vi "sc5511a_reg_write.vi"(0 "deviceHandle":u32 format="%.0x", 2 "Register":T1(ring), 3 "Data In U64":u64 format="%.0x", 5 "error in":errorcluster) -> (14 "deviceHandle":u32 format="%.0x", 19 "error out":errorcluster)   [LabVIEW 2010]
uses:
  sc5511a_rs232.dll
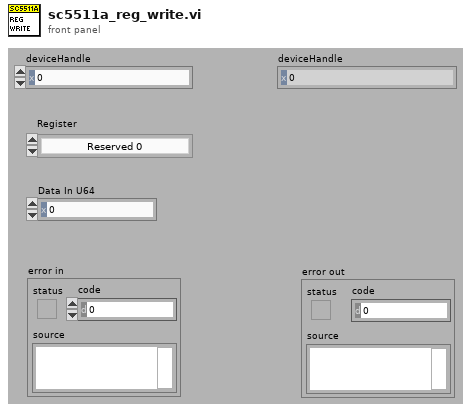
[diagram p1: front panel]
types:
  T1 = enum16{"Reserved 0", "Init", "System Active", "SynthMode", "RF Mode", "List Mode Config", "List Start Freq", "List Stop Freq", "List Step Freq", "List Dwell Time", "List Run Cycles", "Reserved1", "List Buffer Size", "List Buffer Write", "List Buffer to Mem Transfer", "Soft Trigger", "RF Frequency", "RF Level", "RF Enable", "Reserved2", "Auto Level Disable", "ALC Mode", "RF1 Standby", "Reference Setting", "Reference Dac", "ALC Dac", "Reserved3", "Store Default State", "Reserved4", "Reserved5", "RF2 Standby", "RF2 Frequency"}
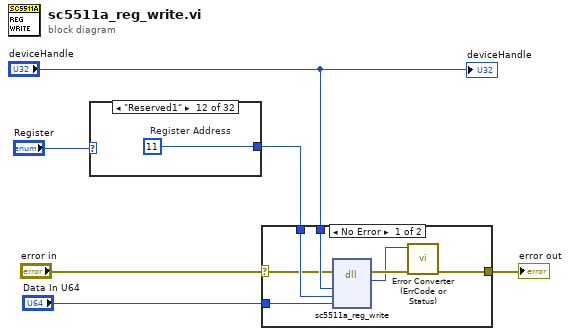
[diagram p0: block diagram]
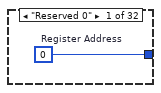
[diagram p2: hidden frame]
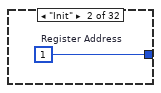
[diagram p3: hidden frame]
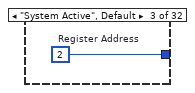
[diagram p4: hidden frame]
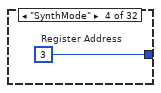
[diagram p5: hidden frame]
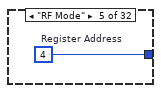
[diagram p6: hidden frame]
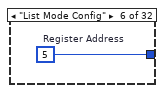
[diagram p7: hidden frame]
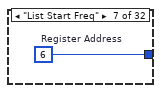
[diagram p8: hidden frame]
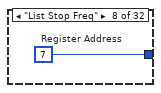
[diagram p9: hidden frame]
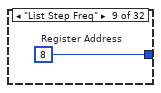
[diagram p10: hidden frame]
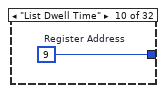
[diagram p11: hidden frame]
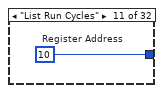
[diagram p12: hidden frame]
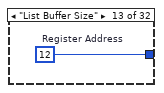
[diagram p13: hidden frame]
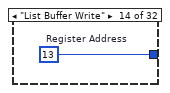
[diagram p14: hidden frame]
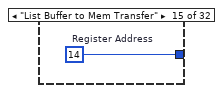
[diagram p15: hidden frame]
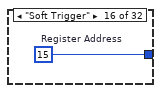
[diagram p16: hidden frame]
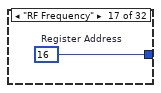
[diagram p17: hidden frame]
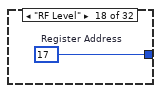
[diagram p18: hidden frame]
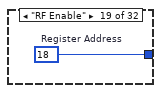
[diagram p19: hidden frame]
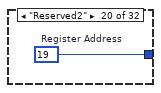
[diagram p20: hidden frame]
diagram:
  n1 = case shown="\"Reserved1\"" "Register" {
    tunnel: [w7 w8 w9 w10 w11 w12 w13 w14 w15 w16 w17 w18 w19 w20 w21 w22 w23 w24 w25 w26 w27 w28 w29 w30 w31 w32 w33 w34 w35 w36 w37 w38] -> w2
    frame "Reserved 0" {
      w7 = u8 0  # Register Address
    }
    frame "Init" {
      w8 = u8 1  # Register Address
    }
    frame "System Active", Default {
      w9 = u8 2  # Register Address
    }
    frame "SynthMode" {
      w10 = u8 3  # Register Address
    }
    frame "RF Mode" {
      w11 = u8 4  # Register Address
    }
    frame "List Mode Config" {
      w12 = u8 5  # Register Address
    }
    frame "List Start Freq" {
      w13 = u8 6  # Register Address
    }
    frame "List Stop Freq" {
      w14 = u8 7  # Register Address
    }
    frame "List Step Freq" {
      w15 = u8 8  # Register Address
    }
    frame "List Dwell Time" {
      w16 = u8 9  # Register Address
    }
    frame "List Run Cycles" {
      w17 = u8 10  # Register Address
    }
    frame "Reserved1" {
      w18 = u8 11  # Register Address
    }
    frame "List Buffer Size" {
      w19 = u8 12  # Register Address
    }
    frame "List Buffer Write" {
      w20 = u8 13  # Register Address
    }
    frame "List Buffer to Mem Transfer" {
      w21 = u8 14  # Register Address
    }
    frame "Soft Trigger" {
      w22 = u8 15  # Register Address
    }
    frame "RF Frequency" {
      w23 = u8 16  # Register Address
    }
    frame "RF Level" {
      w24 = u8 17  # Register Address
    }
    frame "RF Enable" {
      w25 = u8 18  # Register Address
    }
    frame "Reserved2" {
      w26 = u8 19  # Register Address
    }
    frame "Auto Level Disable" {
      w27 = u8 20  # Register Address
    }
    frame "ALC Mode" {
      w28 = u8 21  # Register Address
    }
    frame "RF1 Standby" {
      w29 = u8 22  # Register Address
    }
    frame "Reference Setting" {
      w30 = u8 23  # Register Address
    }
    frame "Reference Dac" {
      w31 = u8 24  # Register Address
    }
    frame "ALC Dac" {
      w32 = u8 25  # Register Address
    }
    frame "Reserved3" {
      w33 = u8 26  # Register Address
    }
    frame "Store Default State" {
      w34 = u8 27  # Register Address
    }
    frame "Reserved4" {
      w35 = u8 28  # Register Address
    }
    frame "Reserved5" {
      w36 = u8 29  # Register Address
    }
    frame "RF2 Standby" {
      w37 = u8 30  # Register Address
    }
    frame "RF2 Frequency" {
      w38 = u8 31  # Register Address
    }
  }
  n2 = case shown="No Error" "error in" {
    selector: "error in" -> [w39 w46]
    tunnel: [w45 w46] -> w5
    tunnel: "Data In U64" -> [w42 _]
    tunnel: "deviceHandle" -> [w41 _]
    tunnel: w2 -> [w40 _]
    frame No Error {
      n3 = dll-call lib="sc5511a_rs232.dll" fn="sc5511a_reg_write"(error in=w39, "deviceHandle"=w41, "Register"=w40, "Data In"=w42) -> (error out=w44:errorcluster, "return type"=w43:i32)  [unwired: 5 in, 1 out]
      n4 = call "Error Converter (ErrCode or Status).vi"("error in (no error)"=w44, "error code"=w43) -> ("error out"=w45:errorcluster)  [unwired: 9 in]
    }
    frame Error {
    }
  }
  "error out" <- w5
  "deviceHandle" <- "deviceHandle"
